vi "myRIO__TCP_constants_byteRange_messageType_quit.vi"() -> (2 "output_Quit_byte":u8=81, 3 "output_Quit_char":string="Q")   [LabVIEW 2014]
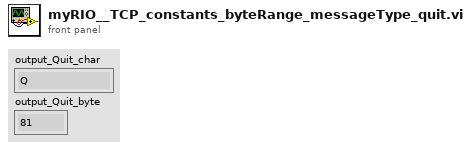
[diagram p1: front panel]
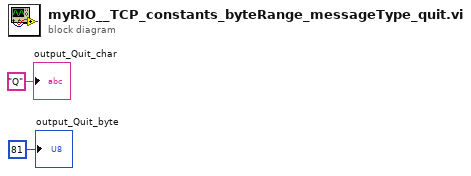
[diagram p0: block diagram]
diagram:
  "output_Quit_char" <- "Q"
  "output_Quit_byte" <- u8 81
